vi "Load Device.vi"(8 "error in (no error)":errorcluster, 9 "device":refnum<class "Device.lvclass">, 10 "Device Manager in":refnum<class "Device Manager.lvclass">, 11 "Caller Actor in":refnum<class "Actor.lvclass">) -> (0 "error out":errorcluster, 2 "Device Manager out":refnum<class "Device Manager.lvclass">, 3 "Caller Actor out":refnum<class "Actor.lvclass">)   [LabVIEW 2020, in "Device Manager.lvclass"]
uses:
  Device Manager.lvclass
  <vilib>/ActorFramework/Actor/Actor.lvclass
  Device/Device/Device.lvclass
  Device/Device Messages/Load Action Msg/Load Action Msg.lvclass
  Device/Device Messages/Configure Action Msg/Configure Action Msg.lvclass
  Device/Device Messages/Start Action Msg/Start Action Msg.lvclass
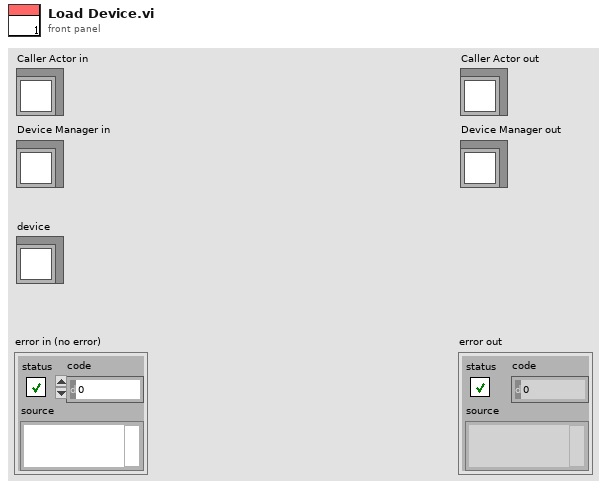
[diagram p1: front panel]
types:
  T1 = map{string, refnum<class "Message Enqueuer.lvclass">}
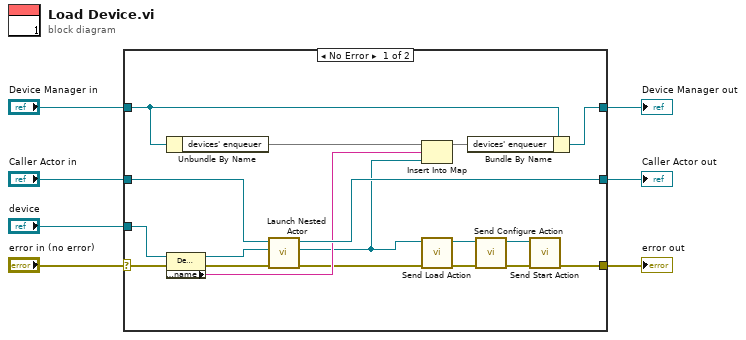
[diagram p0: block diagram]
diagram:
  n1 = case shown="No Error" "error in (no error)" {
    selector: "error in (no error)" -> [w23 w28]
    tunnel: [w8 w28] -> w6
    tunnel: [w17 w27] -> w4
    tunnel: "Device Manager in" -> [w19 w27]
    tunnel: "device" -> [w15 _]
    tunnel: "Caller Actor in" -> [w25 w26]
    tunnel: [w24 w26] -> w1
    frame No Error {
      n2 = Unbundle By Name(w19) -> ("devices' enqueuer"=w21:T1)
      n3 = property class="Device.lvclass"(reference=w15, error in=w23) -> (reference out=w16:refnum<class "Device.lvclass">, error out=w22:errorcluster, "Accessor:name"=w20:string)
      n4 = call <vilib>:"Launch Nested Actor.vi"("error in (no error)"=w22, "Nested Actor"=w16, "Caller Actor in"=w25) -> ("error out"=w14:errorcluster, "Nested Actor's Enqueuer"=w13:refnum<class "Message Enqueuer.lvclass">, "Caller Actor out"=w24:refnum<class "Actor.lvclass">)  [unwired: 6 in]
      n5 = Insert Into Map(map in=w21, key=w20, value=w13) -> (map out=w18:T1)  [unwired: 2 out]
      n6 = call "Send Load Action.vi"("error in (no error)"=w14, "Message Enqueuer"=w13) -> ("error out"=w12:errorcluster, "Message Enqueuer out"=w11:refnum<class "Message Enqueuer.lvclass">)  [unwired: 8 in]
      n7 = Bundle By Name(cluster=w19, "devices' enqueuer"=w18) -> (w17:refnum<class "Device Manager.lvclass">)
      n8 = call "Send Configure Action.vi"("error in (no error)"=w12, "Message Enqueuer"=w11) -> ("error out"=w10:errorcluster, "Message Enqueuer out"=w9:refnum<class "Message Enqueuer.lvclass">)  [unwired: 8 in]
      n9 = call "Send Start Action.vi"("error in (no error)"=w10, "Message Enqueuer"=w9) -> ("error out"=w8:errorcluster)  [unwired: 8 in, 1 out]
    }
    frame Error {
    }
  }
  "error out" <- w6
  "Device Manager out" <- w4
  "Caller Actor out" <- w1
